vi "Untitled 3.vi"() -> ()   [LabVIEW 2018]
uses:
  <vilib>/regexp/Match Regular Expression.xnode
panel:
  out "string":string
  out "concatenated string":string
  out "output 1":i32
  out "substring 2":string
  out "substring":string
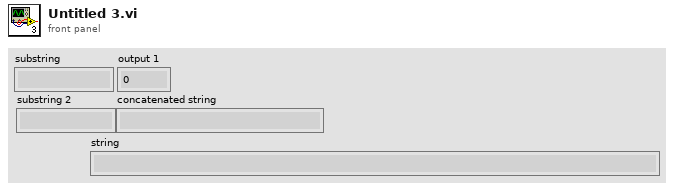
[diagram p1: front panel]
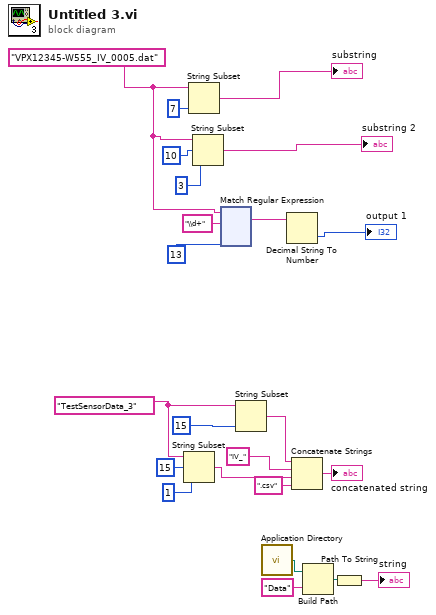
[diagram p0: block diagram]
diagram:
  w8 = "TestSensorData_3" ("string")
  w16 = "VPX12345-W555_IV_0005.dat"
  n1 = String Subset(string=w8, offset (0)=15, length (rest)=1 ("length (rest)")) -> (substring=w7:string)
  n2 = String Subset(string=w16, length (rest)=7 ("length (rest)")) -> (substring=→"substring":string)  [unwired: 1 in]
  n3 = String Subset(string=w16, offset (0)=10, length (rest)=3 ("length (rest)")) -> (substring=→"substring 2":string)
  n4 = xnode "Match Regular Expression"("input string"=w16, "regular expression"="\\d+", "offset (0)"=u32 13 ("initial scan location")) -> ("whole match"=w15:string)  [unwired: 3 in, 4 out]
  n5 = String Subset(string=w8, length (rest)=15 ("length (rest)")) -> (substring=w13:string)  [unwired: 1 in]
  n6 = call <vilib>:"Application Directory.vi"() -> ("Application Directory"=w2:path)
  n7 = Decimal String To Number(string=w15) -> (number=→"output 1":i32)  [unwired: 2 in, 1 out]
  n8 = Concatenate Strings(w13, "IV_" ("string"), w7, ".csv" ("string")) -> (→"concatenated string":string)
  n9 = Build Path(base path=w2, name or relative path="Data") -> (appended path=w3:path)
  n10 = Path To String(path=w3) -> (string=→"string":string)
